vi "Read.vi"(8 "error in (no error)":errorcluster, 9 "timeout ms (25000)":i32, 11 "connection ID":refnum<k5>) -> (0 "error out":errorcluster, 1 "Opcode":u8, 2 "Data":string, 3 "connection ID out":refnum<k5>)   [LabVIEW 2013, in "WebSockets.lvlib"]
doc: "Reads and decodes an incoming WebSockets message."
uses:
  WebSockets.lvlib
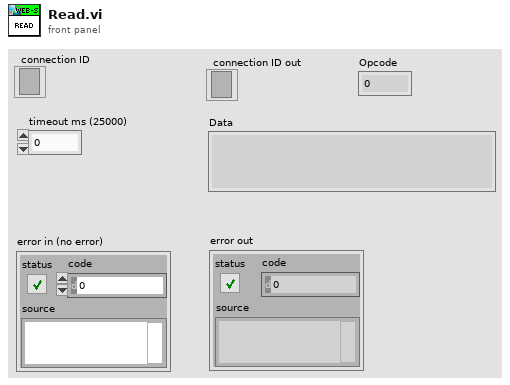
[diagram p1: front panel]
types:
  T1 = enum16{"Standard", "Buffered", "CRLF", "Immediate"}
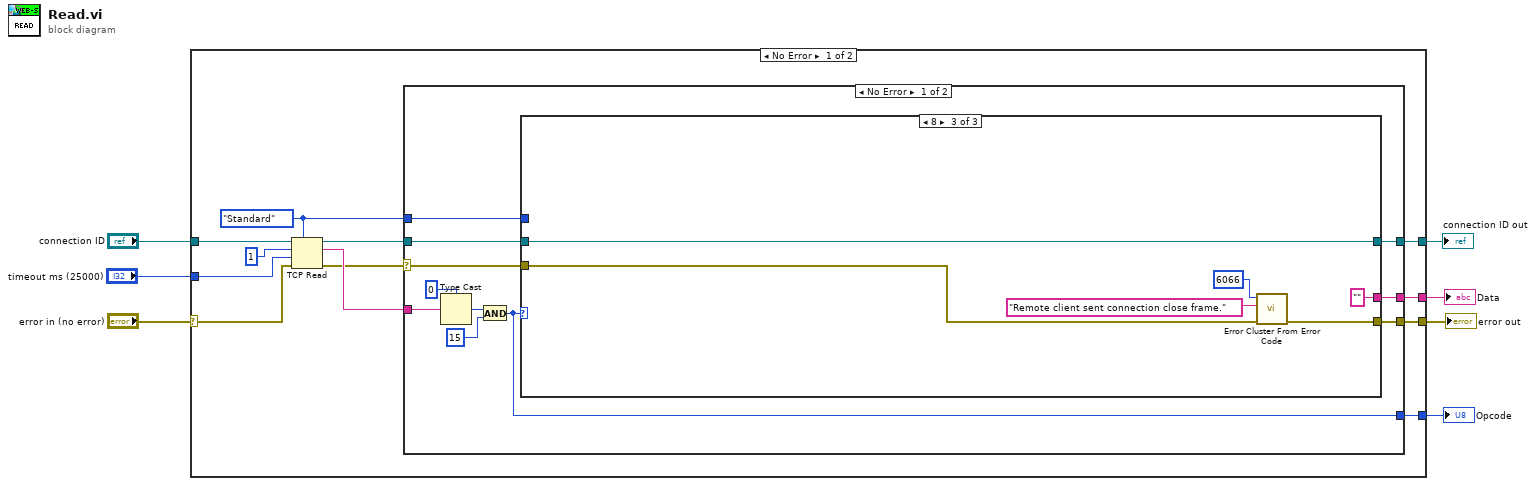
[diagram p0: block diagram]
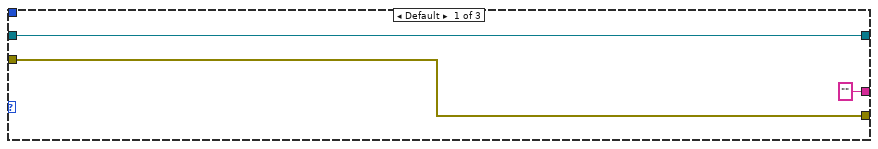
[diagram p2: hidden frame]
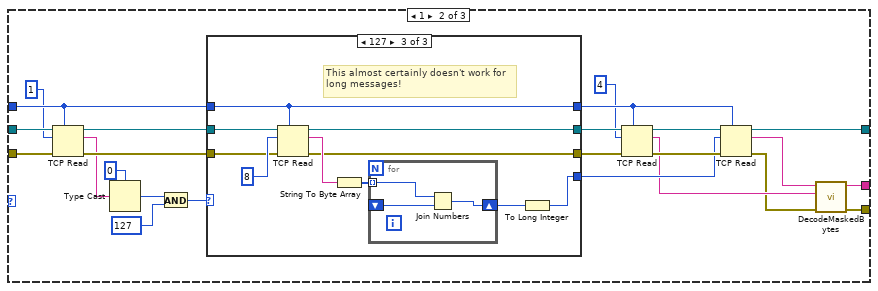
[diagram p3: hidden frame]
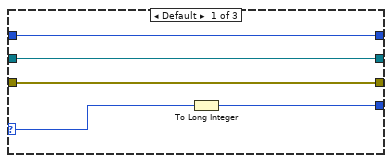
[diagram p4: hidden frame]
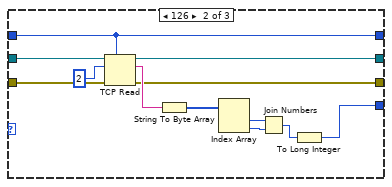
[diagram p5: hidden frame]
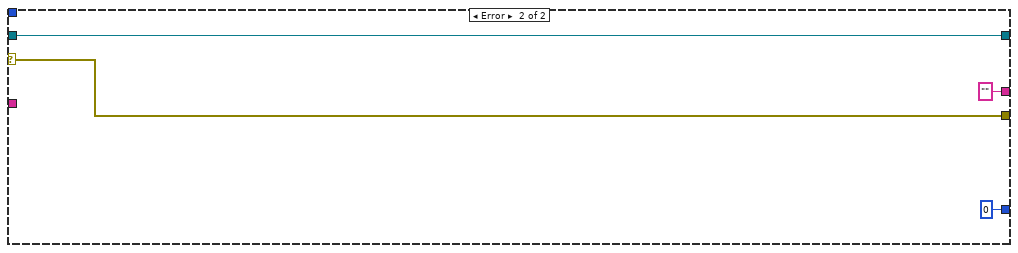
[diagram p6: hidden frame]
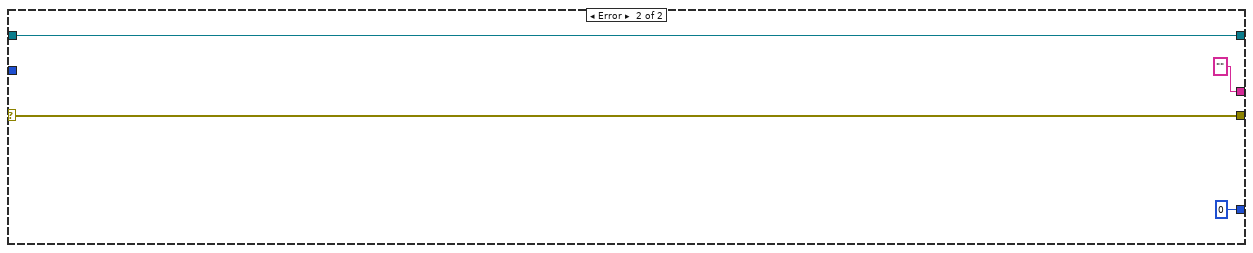
[diagram p7: hidden frame]
diagram:
  n1 = case shown="No Error" "error in (no error)" {
    selector: "error in (no error)" -> [w13 w101]
    tunnel: "connection ID" -> [w19 w100]
    tunnel: [w14 w100] -> w6
    tunnel: [w12 "" ("data out")] -> w5
    tunnel: [w11 w101] -> w3
    tunnel: "timeout ms (25000)" -> [w10 _]
    tunnel: [w8 u8 0] -> w1
    frame No Error {
      w15 = T1."Standard" ("mode (standard)")
      n2 = TCP Read(connection ID=w19, bytes to read=1, error in (no error)=w13, 7:w15, 9:w10) -> (connection ID out=w16:refnum<k5>, data out=w17:string, error out=w9:errorcluster)
      n3 = case shown="No Error" w9 {
        selector: w9 -> [w25 w95]
        tunnel: w17 -> [w24 _]
        tunnel: w16 -> [w30 w97]
        tunnel: w15 -> [w29 _]
        tunnel: [w28 w97] -> w14
        tunnel: [w27 "" ("Decoded Data")] -> w12
        tunnel: [w26 w95] -> w11
        tunnel: [w20 u8 0] -> w8
        frame No Error {
          n4 = Type Cast(type=u8 0 ("element"), x=w24) -> (*(type *) &x=w22:u8)
          n5 = And(x=w22, y=u8 15) -> (x .and. y?=w20:u8)
          n6 = case shown="8" w20 {
            tunnel: w30 -> [w33 w42 w93]
            tunnel: w29 -> [_ w40 _]
            tunnel: [w33 w57 w93] -> w28
            tunnel: ["" ("Decoded Data") w45 "" ("Decoded Data")] -> w27
            tunnel: [w31 w43 w91] -> w26
            tunnel: w25 -> [w31 w38 w90]
            frame Default {
            }
            frame 1 {
              n7 = TCP Read(connection ID=w42, bytes to read=1, error in (no error)=w38, 7:w40) -> (connection ID out=w41:refnum<k5>, data out=w36:string, error out=w37:errorcluster)  [unwired: 1 in]
              n8 = Type Cast(type=u8 0 ("element"), x=w36) -> (*(type *) &x=w35:u8)
              n9 = And(x=w35, y=u8 127) -> (x .and. y?=w55:u8)
              n10 = case shown="127" w55 {
                selector: w55 -> [w61 _ _]
                tunnel: w41 -> [w62 w74 w83]
                tunnel: [w62 w73 w82] -> w54
                tunnel: w40 -> [w59 w65 w75]
                tunnel: [w60 w66 w79] -> w48
                tunnel: [w59 w65 w75] -> w52
                tunnel: [w58 w64 w77] -> w51
                tunnel: w37 -> [w58 w63 w76]
                frame Default {
                  n11 = To Long Integer(number=w61) -> (32bit integer=w60:i32)
                }
                frame 126 {
                  n12 = TCP Read(connection ID=w74, bytes to read=2, error in (no error)=w63, 7:w65) -> (connection ID out=w73:refnum<k5>, data out=w71:string, error out=w64:errorcluster)  [unwired: 1 in]
                  n13 = String To Byte Array(string=w71) -> (unsigned byte array=w70:u8[])
                  n14 = Index Array(array=w70) -> (element #1=w69:u8, element #2=w68:u8)  [unwired: 2 in]
                  n15 = Join Numbers(hi=w69, lo=w68) -> ((hi.lo)=w67:u16)
                  n16 = To Long Integer(number=w67) -> (32bit integer=w66:i32)
                }
                frame 127 {
                  # "This almost certainly doesn't work for long messages!"
                  n17 = TCP Read(connection ID=w83, bytes to read=8, error in (no error)=w76, 7:w75) -> (connection ID out=w82:refnum<k5>, data out=w81:string, error out=w77:errorcluster)  [unwired: 1 in]
                  n18 = String To Byte Array(string=w81) -> (unsigned byte array=w80:u8[])
                  n19 = for {
                    tunnel: w80 -> [w87] mode=indexing
                    shift-right: [w86] -> w78
                    shift-left: _ -> [w85]
                    n20 = Join Numbers(hi=w87, lo=w85) -> ((hi.lo)=w86:u64)
                  }
                  n21 = To Long Integer(number=w78) -> (32bit integer=w79:i32)
                }
              }
              n22 = TCP Read(connection ID=w54, bytes to read=4, error in (no error)=w51, 7:w52) -> (connection ID out=w53:refnum<k5>, data out=w47:string, error out=w50:errorcluster)  [unwired: 1 in]
              n23 = TCP Read(connection ID=w53, bytes to read=w48, error in (no error)=w50, 7:w52) -> (connection ID out=w57:refnum<k5>, data out=w46:string, error out=w44:errorcluster)  [unwired: 1 in]
              n24 = call "DecodeMaskedBytes.vi"("error in (no error)"=w44, "Mask Bytes"=w47, "Encoded Data"=w46) -> ("error out"=w43:errorcluster, "Decoded Data"=w45:string)  [unwired: 7 in]
            }
            frame 8 {
              n25 = call <vilib>:"Error Cluster From Error Code.vi"("error in (no error)"=w90, "error message (\"\")"="Remote client sent connection close frame." ("error message (\"\")"), "error code (0)"=6066) -> ("error out"=w91:errorcluster)  [unwired: 6 in]
            }
          }
        }
        frame Error {
        }
      }
    }
    frame Error {
    }
  }
  "connection ID out" <- w6
  "Data" <- w5
  "error out" <- w3
  "Opcode" <- w1
